vi "Open Actor Core.vi"(8 "error in (no error)":errorcluster, 10 "Actor's Self Q":refnum<class "Message Enqueuer.lvclass">, 11 "Monitor Data":refnum<class "Monitor Data.lvclass">) -> (0 "error out":errorcluster, 2 "Actor Core VI":string)   [LabVIEW 2023, in "Monitored Actor.lvlib" / "Monitor Data.lvclass"]
doc: "Opens the running Actor Core instance for the actor.\n\nIf called in the runtime environoment the Front Panel of the actor core may not be present, so this VI will throw an error.\n\nCopyright: MGI 2016\nAuthor: Derek Trepanier"
uses:
  Monitor Data.lvclass
  builds/Engine/Actor Framework.lvlibp/1abvi3w/vi.lib/ActorFramework/Message Enqueuer/Message Enqueuer.lvclass
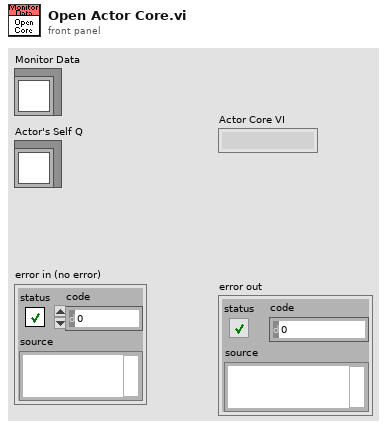
[diagram p1: front panel]
types:
  T1 = typedef "Monitored Actor.lvlib/Monitor Data.lvclass/Actor Data.ctl" = cluster{"Actor Type":string, "Actor Core VI":string, "Self":refnum<class "Message Enqueuer.lvclass">, "Caller":refnum<class "Message Enqueuer.lvclass">, "Actor Label":string, "Last Ping":dbl}
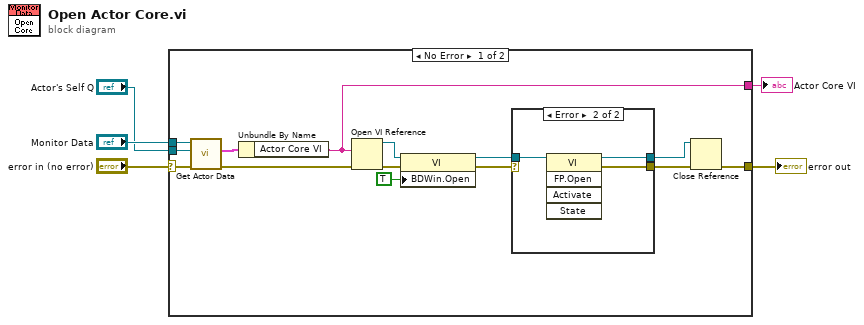
[diagram p0: block diagram]
diagram:
  n1 = case shown="No Error" "error in (no error)" {
    selector: "error in (no error)" -> [w7 w25]
    tunnel: "Monitor Data" -> [w19 _]
    tunnel: "Actor's Self Q" -> [w18 _]
    tunnel: [w9 w25] -> w3
    tunnel: [w6 _] -> w1
    frame No Error {
      n2 = call "Get Actor Data.vi"("error in (no error)"=w7, "Actor's Self Q"=w18, "Monitor Data in"=w19) -> ("error out"=w16:errorcluster, "Actor Data"=w17:T1)  [unwired: 4 in, 3 out]
      n3 = Unbundle By Name(w17) -> ("Actor Core VI"=w6:string)
      n4 = Open VI Reference(vi path=w6, error in (no error)=w16) -> (vi reference=w15:refnum<vi>, error out=w14:errorcluster)  [unwired: 4 in]
      n5 = property class="VI"(reference=w15, error in=w14, "BDWin.Open"=TRUE ("Block Diagram Window:Open")) -> (reference out=w13:refnum<vi>, error out=w12:errorcluster)
      n6 = case shown="Error" w12 {
        selector: w12 -> [w21 _]
        tunnel: w13 -> [w20 w24]
        tunnel: [w20 w23] -> w8
        tunnel: [w21 w22] -> w10
        frame No Error {
        }
        frame Error {
          n7 = invoke class="VI" method="FP.Open"(reference=w24) -> (reference out=w23:refnum<vi>, error out=w22:errorcluster)  [unwired: 4 in, 3 out]
        }
      }
      n8 = Close Reference(reference=w8, error in (no error)=w10) -> (error out=w9:errorcluster)
    }
    frame Error {
    }
  }
  "error out" <- w3
  "Actor Core VI" <- w1
